vi "PointValueMap_ReadWrite_PerformanceTest_I32.vi"() -> ()   [LabVIEW 2017]
uses:
  <vilib>/addons/PointValueMap/subVIs/Point_Read_i32.vi
  <vilib>/addons/PointValueMap/PointValueMap.lvlib
panel:
  in  "Number of Reads":i32=10000
  in  "Number of Writes":i32=10000
  out "Seconds":dbl
  out "Seconds":dbl
  out "Reads/Sec":dbl
  out "Writes/Sec":dbl
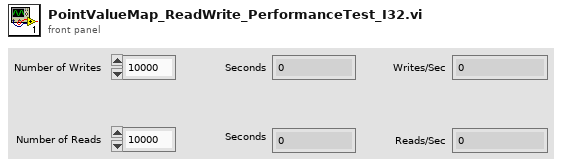
[diagram p1: front panel]
types:
  T1 = typedef "PointValueMap.lvlib/PointMap.ctl" = refnum<data-value>
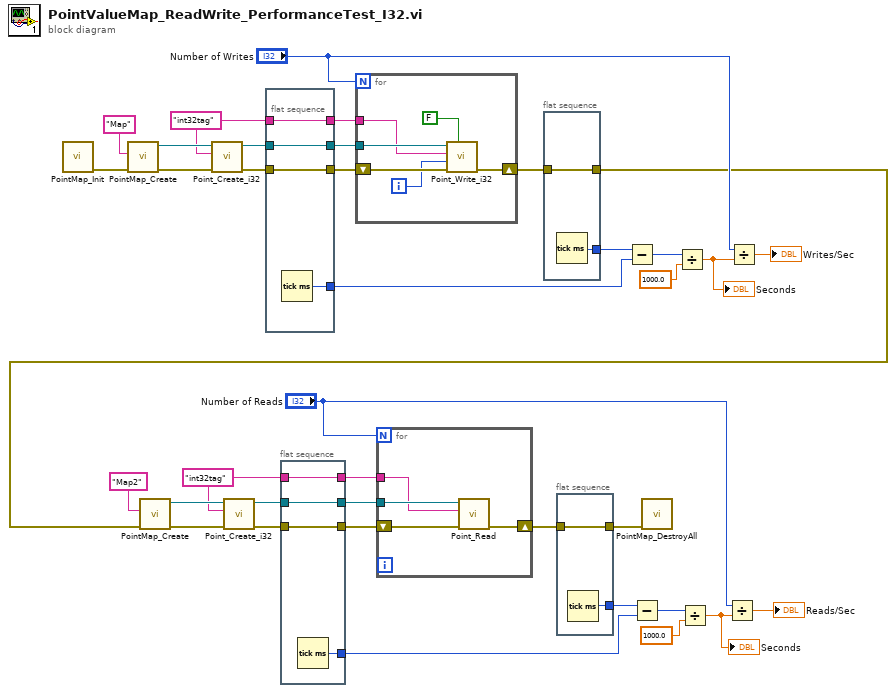
[diagram p0: block diagram]
diagram:
  w4 = "int32tag" ("Tag")
  w6 = "int32tag" ("Tag")
  n1 = call <vilib>:"PointMap_Init.vi"() -> ("error out"=w37:errorcluster)  [unwired: 11 in]
  n2 = call <vilib>:"PointMap_Create.vi"("error in (no error)"=w37, "Name"="Map") -> ("error out"=w34:errorcluster, "Map Out"=w35:T1)  [unwired: 8 in]
  n3 = call <vilib>:"PointMap_Create.vi"("error in (no error)"=w9, "Name"="Map2") -> ("error out"=w12:errorcluster, "Map Out"=w11:T1)  [unwired: 8 in]
  n4 = call <vilib>:"Point_Create_i32.vi"("Error In"=w34, "Tag"=w6, "Map"=w35) -> ("Error Out"=w7:errorcluster, "Map Out"=w32:T1)  [unwired: 7 in]
  n5 = call <vilib>:"Point_Create_i32.vi"("Error In"=w12, "Tag"=w4, "Map"=w11) -> ("Error Out"=w1:errorcluster, "Map Out"=w14:T1)  [unwired: 7 in]
  n6 = flat-sequence {
    tunnel: [w41] -> w33
    tunnel: w32 -> [w41]
    tunnel: [w40] -> w29
    tunnel: [w39] -> w8
    tunnel: w7 -> [w39]
    tunnel: w6 -> [w38]
    tunnel: [w38] -> w5
    frame #0 {
      n7 = Tick Count (ms)() -> (millisecond timer value=w40:u32)
    }
  }
  n8 = flat-sequence {
    tunnel: [w45] -> w13
    tunnel: w14 -> [w45]
    tunnel: [w44] -> w18
    tunnel: w4 -> [w43]
    tunnel: [w43] -> w3
    tunnel: [w42] -> w2
    tunnel: w1 -> [w42]
    frame #0 {
      n9 = Tick Count (ms)() -> (millisecond timer value=w44:u32)
    }
  }
  n10 = for {
    N: "Number of Writes" -> [_]
    tunnel: w33 -> [w51]
    tunnel: w5 -> [w49]
    shift-right: [w48] -> w31
    shift-left: w8 -> [w50]
    i -> [w47]
    n11 = call <vilib>:"Point_Write_i32.vi"("Auto Create?"=FALSE, "Error In"=w50, "Value"=w47, "Tag"=w49, "Map"=w51) -> ("Error Out"=w48:errorcluster)  [unwired: 5 in, 1 out]
  }
  n12 = for {
    N: "Number of Reads" -> [_]
    tunnel: w13 -> [w55]
    tunnel: w3 -> [w53]
    shift-right: [w52] -> w16
    shift-left: w2 -> [w54]
    n13 = call-poly <vilib>:"Point_Read.vi"("Error In"=w54, "Tag"=w53, "Map"=w55) -> ("Error Out"=w52:errorcluster)  [unwired: 3 in, 5 out]
  }
  n14 = flat-sequence {
    tunnel: [w57] -> w9
    tunnel: w31 -> [w57]
    tunnel: [w56] -> w30
    frame #0 {
      n15 = Tick Count (ms)() -> (millisecond timer value=w56:u32)
    }
  }
  n16 = flat-sequence {
    tunnel: [w59] -> w15
    tunnel: w16 -> [w59]
    tunnel: [w58] -> w17
    frame #0 {
      n17 = Tick Count (ms)() -> (millisecond timer value=w58:u32)
    }
  }
  n18 = Subtract(x=w30, y=w29) -> (x-y=w27:u32)
  n19 = Subtract(x=w17, y=w18) -> (x-y=w20:u32)
  n20 = call <vilib>:"PointMap_DestroyAll.vi"("error in (no error)"=w15) -> ()  [unwired: 10 in, 1 out]
  n21 = Divide(x=w27, y=1000.0) -> (x/y=w26:dbl)
  "Seconds" <- w26
  n22 = Divide(x=w20, y=1000.0) -> (x/y=w21:dbl)
  "Seconds" <- w21
  n23 = Divide(x="Number of Reads", y=w21) -> (x/y=→"Reads/Sec":dbl)
  n24 = Divide(x="Number of Writes", y=w26) -> (x/y=→"Writes/Sec":dbl)
